vi "Size Select.vi"(11 "CtlRef":refnum<vi>) -> ()   [LabVIEW 2020, in "MDI ViewManager.lvlib"]
uses:
  MDI ViewManager.lvlib
  <vilib>/Utility/miscctls.llb/LVBoundsTypeDef.ctl
  <vilib>/Utility/miscctls.llb/LVPositionTypeDef.ctl
panel:
  in  "Position":T1
  in  "Dimension":T2={"Width"=96, "Height"=200}
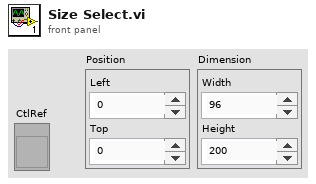
[diagram p1: front panel]
types:
  T1 = typedef "LVPositionTypeDef.ctl" = cluster{"Left":i32, "Top":i32}
  T2 = typedef "LVBoundsTypeDef.ctl" = cluster{"Width":u32, "Height":u32}
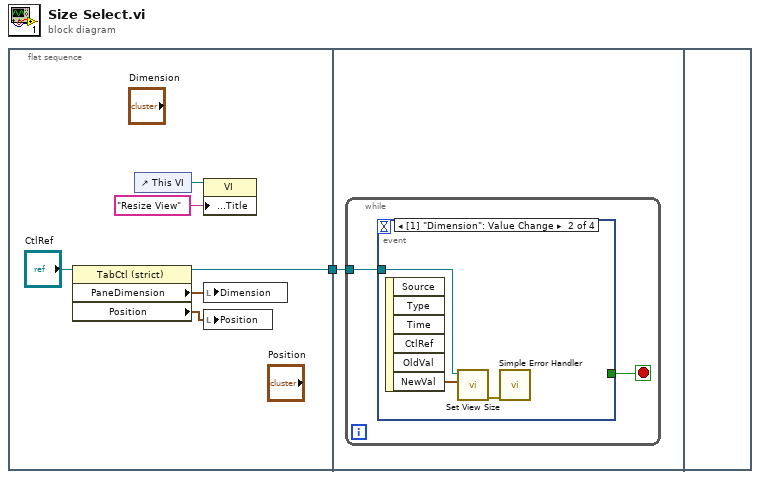
[diagram p0: block diagram]
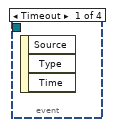
[diagram p2: hidden frame]
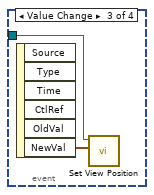
[diagram p3: hidden frame]
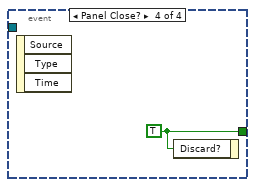
[diagram p4: hidden frame]
diagram:
  n1 = flat-sequence {
    tunnel: [w4] -> w1
    tunnel: w1 -> [w8]
    frame #0 {
      n2 = property class="TabCtl (strict)"(reference="CtlRef") -> (reference out=w4:refnum<vi>, "PaneDimension"=w3:T2, "Position"=w2:T1)  [unwired: 1 in, 1 out]
      n3 = control-ref of="This VI"() -> (w7:refnum<vi>)
      n4 = property class="VI"(reference=w7, "Front Panel.Title"="Resize View" ("VI Name")) -> ()  [unwired: 1 in, 2 out]
      n5 = local write "Dimension"(w3) -> ()
      n6 = local write "Position"(w2) -> ()
    }
    frame #1 {
      n7 = while {
        tunnel: w8 -> [w9]
        stop <- w10 stop-if-true
        n8 = event shown="[1] \"Dimension\": Value Change" {
          selector: _ -> [_ _ _ _]
          dyn-events: _ -> [_ _ _ _]
          timeout: _ -> [_ _ _ _]
          tunnel: [_ _ _ w16] -> w10
          tunnel: w9 -> [_ w13 w15 _]
          event Timeout {
            n9 = event-data() -> ()  [unwired: 1 in, 3 out]
          }
          event Value Change {
            n10 = event-data() -> ("NewVal"=w11:T2)  [unwired: 1 in, 5 out]
            n11 = call "Set View Size.vi"("TabDimension"=w11, "TabControlRef in"=w13) -> ("error out"=w12:errorcluster)  [unwired: 8 in, 1 out]
            n12 = call <vilib>:"Simple Error Handler.vi"("error in (no error)"=w12) -> ()  [unwired: 4 in, 5 out]
          }
          event Value Change {
            n13 = event-data() -> ("NewVal"=w14:T1)  [unwired: 1 in, 5 out]
            n14 = call "Set View Position.vi"("Position"=w14, "TabControlRef in"=w15) -> ()  [unwired: 8 in, 2 out]
          }
          event Panel Close? {
            w16 = TRUE ("Discard?")
            n15 = event-data() -> ()  [unwired: 1 in, 3 out]
            n16 = event-data("Discard?"=w16) -> ()  [unwired: 1 in, 1 out]
          }
        }
      }
    }
    frame #2 {
    }
  }
